vi "Global 1.vi"() -> ()   [LabVIEW 2014]
panel:
  in  "turn":dbl
  in  "power":dbl
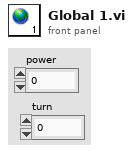
[diagram p1: front panel]
diagram:
